vi "TableScroller.vi"(0 "TableRef":refnum<vi>, 7 "InsertedRow":i32, 11 "#ofRows":i32) -> ()   [LabVIEW 2013]
uses:
  <vilib>/Utility/miscctls.llb/LVRowAndColumnTypeDef.ctl
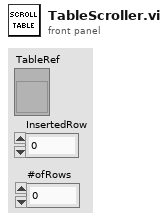
[diagram p1: front panel]
types:
  T1 = typedef "LVRowAndColumnTypeDef.ctl" = cluster{"Row":i32, "Column":i32}
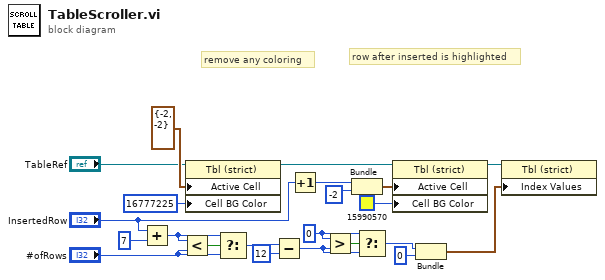
[diagram p0: block diagram]
diagram:
  w18 = 0 ("y")
  # "row after inserted is highlighted"
  # "remove any coloring"
  n1 = Add(x="InsertedRow", y=7) -> (x+y=w1:i32)
  n2 = Less?(x=w1, y="#ofRows") -> (x < y?=w22:bool)
  n3 = property on="Property Node" class="Tbl (strict)"(reference="TableRef", "Active Cell"=T1 {"Row"=-2, "Column"=-2} ("Active Cell:Active Cell"), "Cell BG Color"=u32 16777225 ("Active Cell:Cell Background Color")) -> (reference out=w10:refnum<vi>)  [unwired: 1 in, 1 out]
  n4 = Select(t=w1, s=w22, f="#ofRows") -> (s? t:f=w16:i32)
  n5 = Subtract(x=w16, y=12) -> (x-y=w19:i32)
  n6 = Increment(x="InsertedRow") -> (x+1=w5:i32)
  n7 = Greater?(x=w18, y=w19) -> (0:w20:bool)
  n8 = Bundle(w5, -2) -> (w13:cluster{i32, i32})  [unwired: 1 in]
  n9 = Select(t=w18, s=w20, f=w19) -> (s? t:f=w3:i32)
  n10 = property on="Property Node" class="Tbl (strict)"(reference=w10, "Active Cell"=w13, "Cell BG Color"=u32 15990570) -> (reference out=w6:refnum<vi>)  [unwired: 1 in, 1 out]
  n11 = Bundle("y"=w3, "y"=0) -> (w21:cluster{"y":i32, "y":i32})  [unwired: 1 in]
  n12 = property on="Property Node" class="Tbl (strict)"(reference=w6, "Index Values"=w21) -> ()  [unwired: 1 in, 2 out]
